vi "observator.vi"(0 "d_t":dbl, 1 "e_x":dbl, 2 "e_y":dbl) -> (3 "observation":dbl[](array[numeric]), 4 "scaled_obs":dbl[](array[numeric]), 5 "scaled_obs_x":dbl[](array[numeric]), 6 "scaled_obs_y":dbl[](array[numeric]))   [LabVIEW 2019]
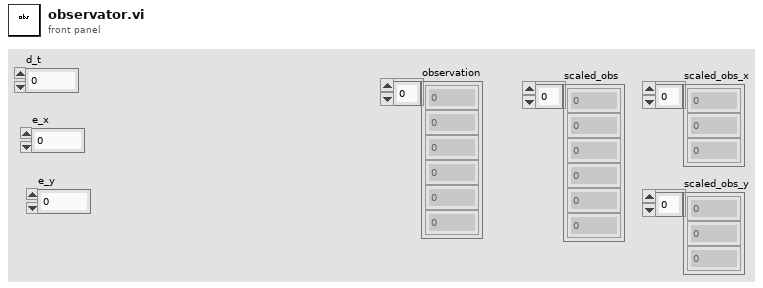
[diagram p1: front panel]
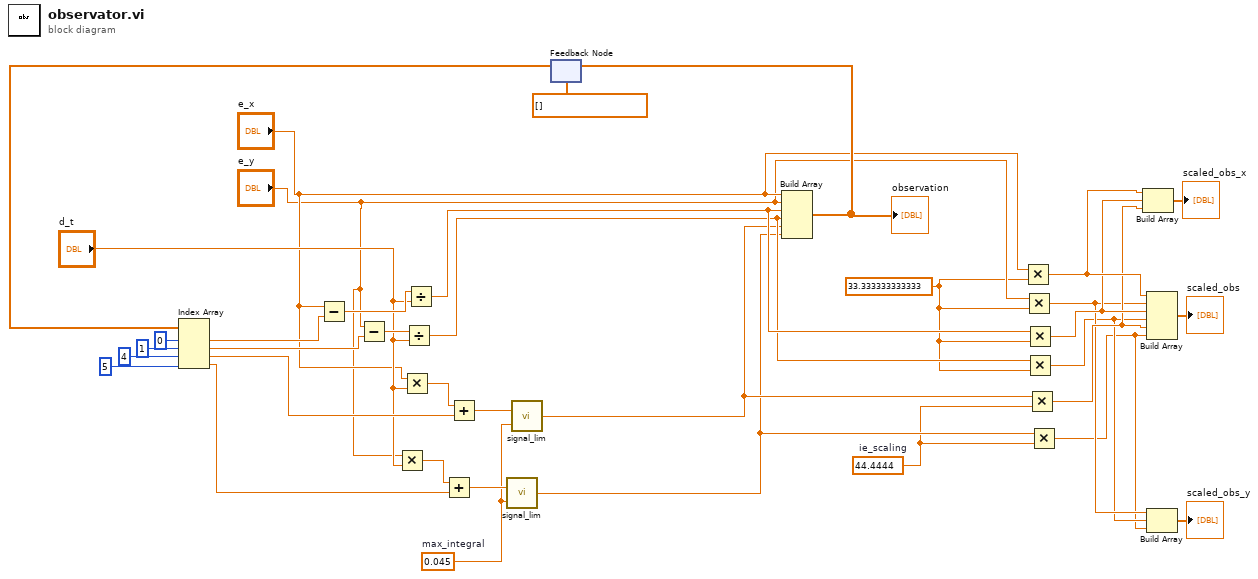
[diagram p0: block diagram]
diagram:
  w11 = 44.4444  # ie_scaling
  w10 = 33.333333333333
  w24 = 0.045  # max_integral
  n1 = Multiply(x="e_y", y="d_t") -> (x*y=w26:dbl)
  n2 = Multiply(x="e_x", y="d_t") -> (x*y=w28:dbl)
  n3 = feedback #1(dbl[] []) -> (w18:dbl[])
  n4 = Index Array(array=w18, index #1=0 ("index"), index #2=1 ("index"), index #3=4 ("index"), index #4=5 ("index")) -> (element #1=w32:dbl, element #2=w30:dbl, element #3=w23:dbl, element #4=w22:dbl)
  n5 = Subtract(x="e_x", y=w32) -> (x-y=w31:dbl)
  n6 = Subtract(x="e_y", y=w30) -> (x-y=w29:dbl)
  n7 = Divide(x=w29, y="d_t") -> (x/y=w14:dbl)
  n8 = Divide(x=w31, y="d_t") -> (x/y=w15:dbl)
  n9 = Add(x=w26, y=w22) -> (x+y=w25:dbl)
  n10 = Add(x=w28, y=w23) -> (x+y=w27:dbl)
  n11 = call "signal_lim.vi"("lim"=w24, "x"=w25) -> ("y"=w12:dbl)
  n12 = call "signal_lim.vi"("lim"=w24, "x"=w27) -> ("y"=w13:dbl)
  n13 = Build Array("e_x", "e_y", w15, w14, w13, w12) -> (w20:dbl[])
  "observation" <- w20
  n14 = feedback-in #1(w20) -> ()
  n15 = Multiply(x="e_x", y=w10) -> (x*y=w8:dbl)
  n16 = Multiply(x="e_y", y=w10) -> (x*y=w5:dbl)
  n17 = Multiply(x=w15, y=w10) -> (x*y=w7:dbl)
  n18 = Multiply(x=w14, y=w10) -> (x*y=w4:dbl)
  n19 = Multiply(x=w13, y=w11) -> (x*y=w6:dbl)
  n20 = Multiply(x=w12, y=w11) -> (x*y=w3:dbl)
  n21 = Build Array(w8, w7, w6) -> (→"scaled_obs_x":dbl[])
  n22 = Build Array(w8, w5, w7, w4, w6, w3) -> (→"scaled_obs":dbl[])
  n23 = Build Array(w5, w4, w3) -> (→"scaled_obs_y":dbl[])
